vi "New Extract Lines on Grass.vi"(7 "error in":errorcluster) -> (27 "error out":errorcluster)   [LabVIEW 2009]
uses:
  <vilib>/vision/NI_Vision_Development_Module.lvlib
panel:
  out "Image Out":T1(plugin-control)
  out "Histogram Graph":u32[][](graph)
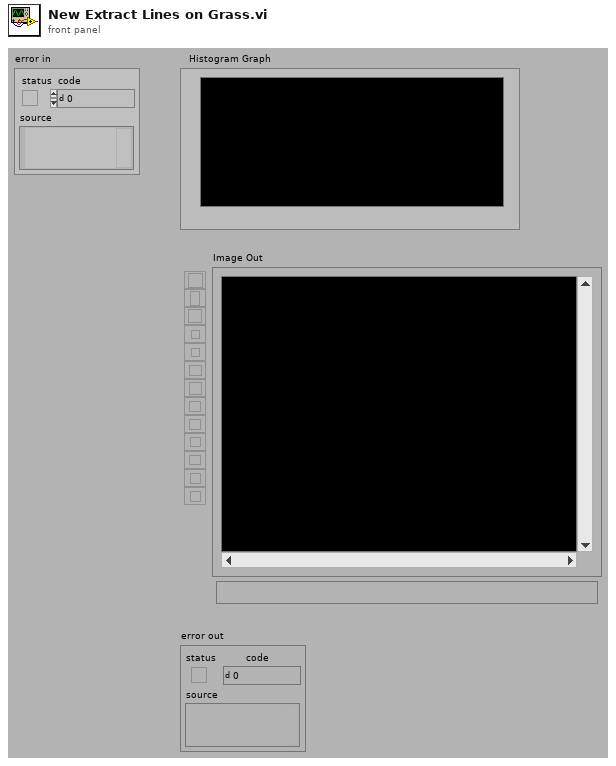
[diagram p1: front panel]
types:
  T1 = typedef "IMAQ Image.ctl" = refnum<image>
  T2 = cluster{"Global Rectangle":i32[], "Contours":cluster{"ID":enum32{"External", "Internal"}, "Type":u32, "Coordinates":i32[]}[]}[]
  T3 = cluster{"Global Rectangle":i32[], "Contours":cluster{"ID":enum32{"External", "Internal"}, "Type":u32, "Coordinates":i32[]}[]}
  T4 = typedef "Image Type" = u32
  T5 = cluster{"Minimal Value":sgl, "Maximal Value":sgl, "Mean Value":sgl, "Standard  Variation":sgl, "Area (pixels)":i32}
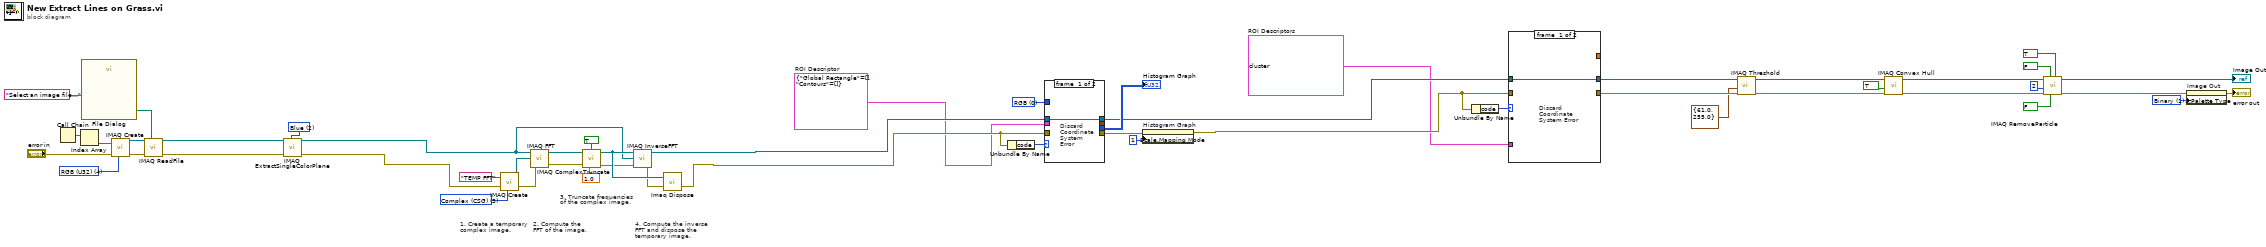
[diagram p0: block diagram]
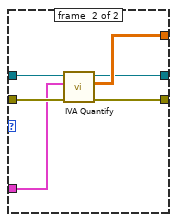
[diagram p2: hidden frame]
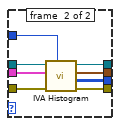
[diagram p3: hidden frame]
diagram:
  w2 = u32 1 items=["Grayscale", "Binary", "Gradient", "Rainbow", "Temperature", "User Defined"] ("Palette")
  w17 = T2 [{"Global Rectangle"=[0, 0, 160, 120], "Contours"=[{"ID"=enum."External", "Type"=3, "Coordinates"=[0, 0, 160, 120]}]}]  # ROI Descriptors
  w24 = u16 0 items=["RGB", "HSL", "HSV", "HSI"] ("Color Mode")
  w22 = T3 {"Global Rectangle"=[], "Contours"=[]}  # ROI Descriptor
  w28 = T4 3 items=["Grayscale (U8)", "Grayscale (I16)", "Grayscale (SGL)", "Complex (CSG)", "RGB (U32)", "HSL (U32)", "RGB (U64)", "Grayscale (U16)"] ("Image Type")
  w43 = 2 items=["Red", "Green", "Blue", "Hue", "Saturation", "Luminance", "Value", "Intensity"] ("Color Plane")
  w44 = T4 4 items=["Grayscale (U8)", "Grayscale (I16)", "Grayscale (SGL)", "Complex (CSG)", "RGB (U32)", "HSL (U32)", "RGB (U64)", "Grayscale (U16)"] ("Image Type")
  # "4. Compute the inverse\nFFT and dispose the\ntemporary image."
  # "3. Truncate frequencies\nof the complex image."
  # "2. Compute the\nFFT of the image."
  # "1. Create a temporary\ncomplex image."
  n1 = Call Chain() -> (call chain=w48:string[])
  n2 = Index Array(array=w48) -> (element=w47:string)  [unwired: 1 in]
  n3 = call "File Dialog"("prompt"="Select an image file...") -> ("selected path"=w45:path)  [unwired: 6 in, 8 out]
  n4 = call "IMAQ Create"("Image Name"=w47, "Image Type"=w44, "error in (no error)"="error in") -> ("New Image"=w51:T1, "error out"=w50:errorcluster)  [unwired: 1 in, 1 out]
  n5 = call "IMAQ ReadFile"("File Path"=w45, "error in (no error)"=w50, "Image"=w51) -> ("error out"=w52:errorcluster, "Image Out"=w42:T1)  [unwired: 2 in, 5 out]
  n6 = call "IMAQ ExtractSingleColorPlane"("Color Plane"=w43, "error in (no error)"=w52, "Image Src"=w42) -> ("error out"=w41:errorcluster, "Image Dst Out"=w31:T1)  [unwired: 1 in, 6 out]
  n7 = call "IMAQ Create"("Image Name"="TEMP FFT", "Image Type"=w28, "error in (no error)"=w41) -> ("New Image"=w39:T1, "error out"=w32:errorcluster)  [unwired: 1 in, 1 out]
  n8 = call "IMAQ FFT"("error in (no error)"=w32, "Image Dst"=w39, "Image Src"=w31) -> ("error out"=w37:errorcluster, "Image Dst Out"=w38:T1)  [unwired: 1 out]
  n9 = call "IMAQ ComplexTruncate"("error in (no error)"=w37, "Truncation Frequency %"=sgl 1.0, "Image Src"=w38, "Low pass/High pass (Low pass)"=TRUE) -> ("error out"=w35:errorcluster, "Image Dst Out"=w36:T1)  [unwired: 1 in, 2 out]
  n10 = call "IMAQ InverseFFT"("error in (no error)"=w35, "Image Dst"=w31, "Image Src"=w36) -> ("error out"=w34:errorcluster, "Image Dst Out"=w27:T1)  [unwired: 1 out]
  n11 = call "Imaq Dispose"("Image"=w36, "error in (no error)"=w34) -> ("error out"=w33:errorcluster)  [unwired: 1 in, 3 out]
  n12 = Unbundle By Name(w33) -> ("code"=w20:i32)
  n13 = case shown="Default" w20 {
    tunnel: w33 -> [_ w61]
    tunnel: w27 -> [w53 w60]
    tunnel: [_ w59] -> _
    tunnel: [_ w58] -> w25
    tunnel: w24 -> [_ w57]
    tunnel: [_ w56] -> w23
    tunnel: w22 -> [_ w55]
    tunnel: [w53 w54] -> w19
    frame #0 {
      # "Discard\nCoordinate\nSystem\nError"
    }
    frame #1 {
      n14 = call <vilib>:"IVA Histogram.vi"("Color Mode"=w57, "error in (no error)"=w61, "ROI Descriptor"=w55, "Image In"=w60) -> ("error out"=w58:errorcluster, "Histograms"=w56:u32[][], "Statistics"=w59:T5, "Image Out"=w54:T1)  [unwired: 4 out]
    }
  }
  "Histogram Graph" <- w23
  n15 = property on="Histogram Graph"(error in=w25, "Y Scale.Mapping Mode"=u8 1) -> (error out=w21:errorcluster)  [unwired: 1 in, 1 out]
  n16 = Unbundle By Name(w21) -> ("code"=w16:i32)
  n17 = case shown="Default" w16 {
    tunnel: [_ w68] -> _
    tunnel: w19 -> [w62 w67]
    tunnel: w21 -> [_ w66]
    tunnel: [w62 w65] -> w14
    tunnel: [_ w64] -> w18
    tunnel: w17 -> [_ w63]
    frame #0 {
      # "Discard\nCoordinate\nSystem Error"
    }
    frame #1 {
      n18 = call <vilib>:"IVA Quantify.vi"("error in (no error)"=w66, "ROI Descriptors"=w63, "Image"=w67) -> ("error out"=w64:errorcluster, "Results"=w68:sgl[][], "Image Out"=w65:T1)  [unwired: 6 out]
    }
  }
  n19 = call "IMAQ Threshold"("error in (no error)"=w18, "Range"=cluster{"Lower value":sgl, "Upper value":sgl} {"Lower value"=61.0, "Upper value"=255.0}, "Image Src"=w14) -> ("error out"=w13:errorcluster, "Image Dst Out"=w12:T1)  [unwired: 3 in, 4 out]
  n20 = call "IMAQ Convex Hull"("error in (no error)"=w13, "Connectivity 4/8 (8)"=TRUE, "Image Src"=w12) -> ("error out"=w10:errorcluster, "Image Dst Out"=w5:T1)  [unwired: 1 in, 6 out]
  n21 = call "IMAQ RemoveParticle"("Connectivity 4/8 (8)"=TRUE, "Low Pass/High Pass (Low)"=FALSE, "Square/Hexa (Square)"=FALSE, "error in (no error)"=w10, "Number of Erosion"=2, "Image Src"=w5) -> ("error out"=w4:errorcluster, "Image Dst Out"=→"Image Out":T1)  [unwired: 1 in, 3 out]
  n22 = property on="Image Out" class="ImageControl"(error in=w4, "Palette:Palette Type"=w2) -> (error out=→"error out":errorcluster)  [unwired: 1 in, 1 out]
